vi "Mem_SGLArray.vi"(8 "error in (no error)":errorcluster, 11 "dataInfo":T1) -> (0 "error out":errorcluster, 2 "DataPoints":sgl[](array[numeric]))   [LabVIEW 2019, in "Memory Data Access.lvlib"]
uses:
  Memory Data Access.lvlib
  Typedef/memoryDataBlock.ctl
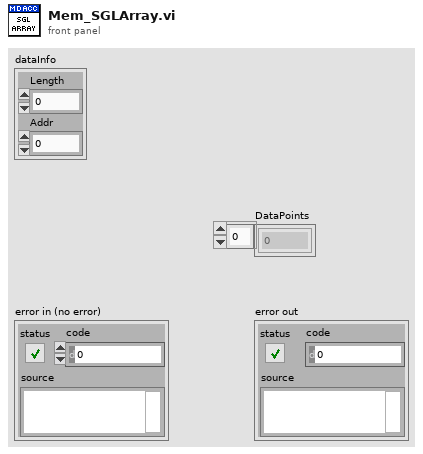
[diagram p1: front panel]
types:
  T1 = typedef "Memory Data Access.lvlib/memoryDataBlock.ctl" = cluster{"Length":u32, "Addr":u64}
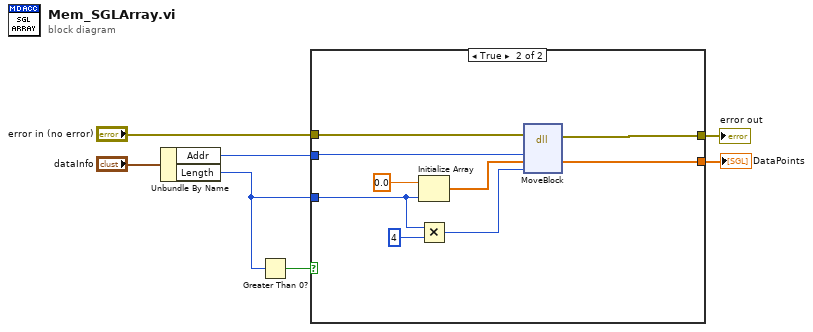
[diagram p0: block diagram]
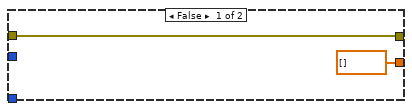
[diagram p2: hidden frame]
diagram:
  n1 = Unbundle By Name("dataInfo") -> ("Addr"=w2:u64, "Length"=w1:u32)
  n2 = Greater Than 0?(x=w1) -> (x > 0?=w5:bool)
  n3 = case shown="True" w5 {
    tunnel: "error in (no error)" -> [w9 w18]
    tunnel: [w9 w17] -> w6
    tunnel: w2 -> [_ w11]
    tunnel: w1 -> [_ w12]
    tunnel: [sgl[] [] ("Destination") w10] -> w4
    frame False {
    }
    frame True {
      n4 = Initialize Array(sgl 0.0, w12) -> (w15:sgl[])
      n5 = Multiply(x=w12, y=u32 4) -> (x*y=w13:u32)
      n6 = dll-call lib="LabVIEW" fn="MoveBlock"(error in=w18, "Address"=w11, "Destination"=w15, "Size"=w13) -> (error out=w17:errorcluster, "Destination"=w10:sgl[])  [unwired: 5 in, 1 out]
    }
  }
  "error out" <- w6
  "DataPoints" <- w4
